vi "ChangeOverTime.vi"(11 "InputNum":dbl) -> (3 "ChangeOverTime":dbl)   [LabVIEW 2020]
doc: "Calulates Change/Time for Input as its given. IF we ever geta divide by zero error it outputs 0 speed"
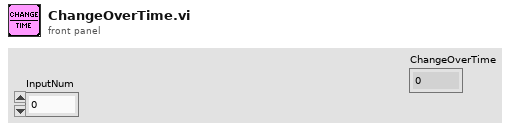
[diagram p1: front panel]
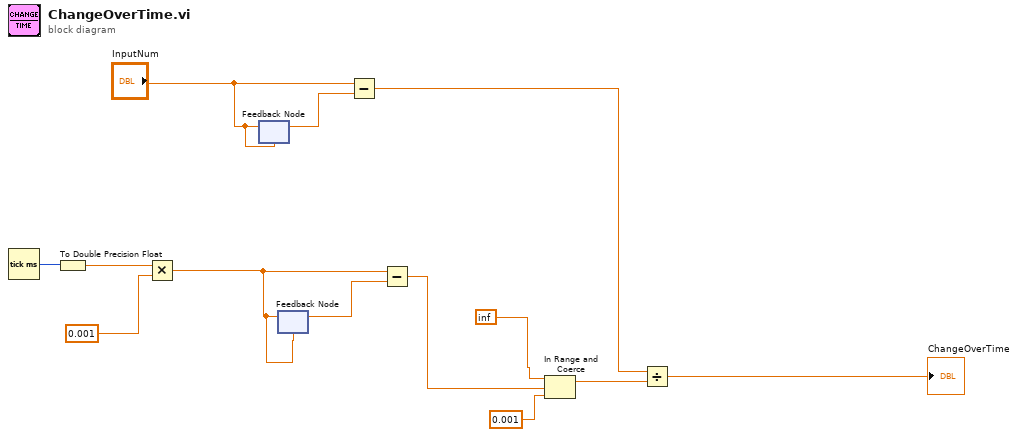
[diagram p0: block diagram]
diagram:
  n1 = Tick Count (ms)() -> (millisecond timer value=w12:u32)
  n2 = To Double Precision Float(number=w12) -> (double precision float=w6:dbl)
  n3 = Multiply(x=w6, y=0.001) -> (x*y=w5:dbl)
  n4 = feedback #1("InputNum") -> (w8:dbl)
  n5 = feedback-in #1("InputNum") -> ()
  n6 = feedback-in #2(w5) -> ()
  n7 = feedback #2(w5) -> (w11:dbl)
  n8 = Subtract(x="InputNum", y=w8) -> (x-y=w10:dbl)
  n9 = Subtract(x=w5, y=w11) -> (x-y=w3:dbl)
  n10 = In Range and Coerce(upper limit=inf, x=w3, lower limit=0.001) -> (coerced(x)=w1:dbl)  [unwired: 1 out]
  n11 = Divide(x=w10, y=w1) -> (x/y=→"ChangeOverTime":dbl)
